vi "DATE-DT Byte Stream to Timestamp.vi"(8 "error in (no error)":errorcluster, 10 "Byte Stream":u8[](array[numeric])) -> (0 "error out":errorcluster, 2 "Value":timestamp)   [LabVIEW 2018, in "TwinCAT ADS.lvclass"]
uses:
  TwinCAT ADS.lvclass
  c220fc55-106a-42bf-a87c-9fb329dce798.vi
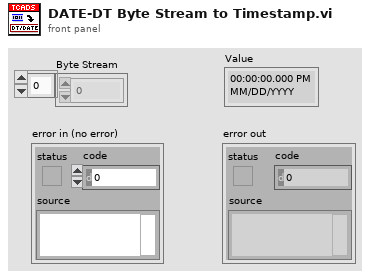
[diagram p1: front panel]
types:
  T1 = typedef "LVDateTimeRec.ctl" = cluster{"fractional second":dbl, "second":i32, "minute":i32, "hour":i32, "day of month":i32, "month":i32, "year":i32, "day of week":i32, "day of year":i32, "DST":i32}
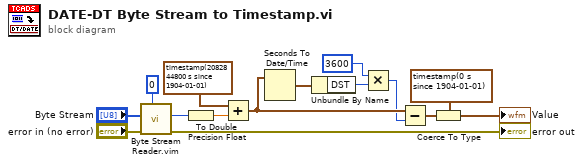
[diagram p0: block diagram]
diagram:
  n1 = call "Byte Stream Reader.vim"("Type"=u32 0, "error in (no error)"="error in (no error)", "Byte Stream"="Byte Stream") -> ("error out"=→"error out":errorcluster, "Value"=w3:u32)  [unwired: 7 in]
  n2 = To Double Precision Float(number=w3) -> (double precision float=w15:dbl)
  n3 = Add(x=timestamp(2082844800 s since 1904-01-01) ("time stamp"), y=w15) -> (x+y=w13:timestamp)
  n4 = Seconds To Date/Time(time stamp (now)=w13) -> (date time rec=w12:T1)  [unwired: 1 in]
  n5 = Unbundle By Name(w12) -> ("DST"=w11:i32)
  n6 = Multiply(x=3600, y=w11) -> (x*y=w9:i32)
  n7 = Subtract(x=w13, y=w9) -> (x-y=w7:timestamp)
  n8 = Coerce To Type(0:w7, 1:timestamp(0 s since 1904-01-01)) -> (2:→"Value":timestamp)
